vi "AH 2700 Dev Mode.vi"() -> ()   [LabVIEW 2019]
doc: "This example shows how to configure the bridge,initiate deviation mode and continuous capacitance measurement, read the results from the bridge, and parse the measurement results."
uses:
  Andeen-Hagerling 2700(400 firmware).lvlib
panel:
  out "Attentap":string
  out "Voltage":dbl
  out "Loss Greater Than":string
  out "Frequency":dbl
  out "Sample Switch":i32
  in  "Dev Average (s)":dbl=0.1 min=0.0 max=999999.9
  out "Loss Chart":dbl(graph)
  out "Capacitance Chart":dbl(graph)
  in  "Aout Bound\nLower Loss (V)":dbl=-10.0 min=-160.0 max=160.0 format="%#_6f"
  in  "Aout Bound\nLower Cap (V)":dbl=-10.0 min=-160.0 max=160.0 format="%#_6f"
  in  "Aout Bound\nUpper Loss (V)":dbl=10.0 min=-160.0 max=160.0 format="%#_6f"
  in  "Aout Bound\nUpper Cap (V)":dbl=10.0 min=-160.0 max=160.0 format="%#_6f"
  out "Loss":dbl format="%#_10f"
  out "Capacitance":dbl format="%#_10f"
  out "Error Message":string
  in  "Dev Point Loss (jpF)":dbl min=-1900.0 max=19000.0 format="%#_10f"
  in  "Dev Point Cap (pF)":dbl=100.0 min=-165000.0 max=1650000.0 format="%#_10f"
  in  "Deviation Margin":dbl=1.0 min=1.0 max=20.0
  in  "Dev Bound\nLower Loss (jpF)":dbl=-0.1 min=-1900.0 max=19000.0 format="%#_6f"
  in  "Dev Bound\nLower Cap (pF)":dbl=99.0 min=-165000.0 max=1650000.0 format="%#_6f"
  in  "Dev Bound\nUpper Loss (jpF)":dbl=0.1 min=-1900.0 max=19000.0 format="%#_6f"
  in  "Dev Bound\nUpper Cap (pF)":dbl=101.0 min=-165000.0 max=1650000.0 format="%#_6f"
  in  "stop":bool
  in  "Bridge\nFrequency (Hz)":dbl(ring)=1000.0 items=["50"=50.0, "60"=60.0, "70"=70.0, "80"=80.0, "100"=100.0, "120"=120.0, "140"=140.0, "160"=160.0, "200"=200.0, "240"=240.0, "300"=300.0, "400"=400.0, "500"=500.0, "600"=600.0, "700"=700.0, "800"=800.0, "1000"=1000.0, "1200"=1200.0, "1400"=1400.0, "1600"=1600.0, "2000"=2000.0, "2400"=2400.0, "3000"=3000.0, "4000"=4000.0, "5000"=5000.0, "6000"=6000.0, "7000"=7000.0, "8000"=8000.0, "10000"=10000.0, "12000"=12000.0, "14000"=14000.0, "16000"=16000.0, "20000"=20000.0]
  in  "Maximum\nVoltage (V)":dbl=15.0 min=0.0003 max=15.0 step=1.0 format="%#.6f"
  in  "Average\nExponent":u16=4 max=15
  in  "VISA resource":refnum<visa-resource-name>
  in  "Serial Configuration":T1={"Baud Rate"=9600, "Parity"=0, "Data Bits"=8, "Stop Bits"=10} {"Stop Bits" items=["1.0"=10, "1.5"=15, "2.0"=20]; "Data Bits" items=["7"=7, "8"=8]; "Parity" items=["None", "Odd", "Even", "Mark", "Space"]; "Baud Rate" items=["300"=300, "600"=600, "1200"=1200, "2400"=2400, "4800"=4800, "9600"=9600, "19200"=19200, "38400"=38400, "57600"=57600, "115200"=115200]}
  # "AH 2700A ULTRA-PRECISION 50Hz-20kHz CAPACITANCE BRIDGE"
  # "Deviation Mode / Analog Out"
  # "Deviation Parameters"
  # "Measurement Parameters"
  # "Analog Out Parameters"
  # "Measurement Results"
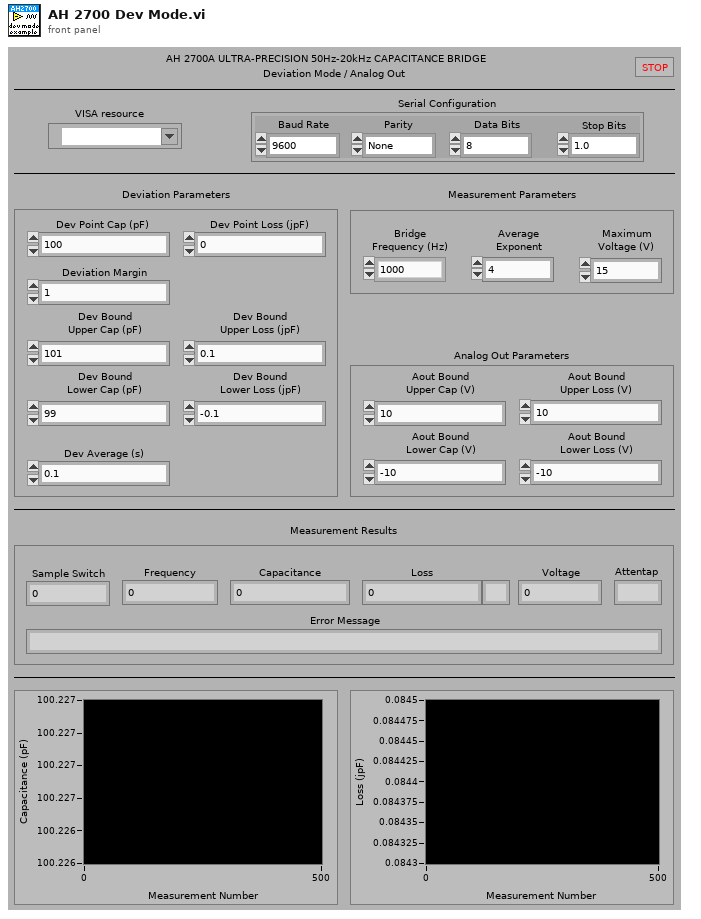
[diagram p1: front panel]
types:
  T1 = cluster{"Baud Rate":u32, "Parity":u16, "Data Bits":u16, "Stop Bits":u16}
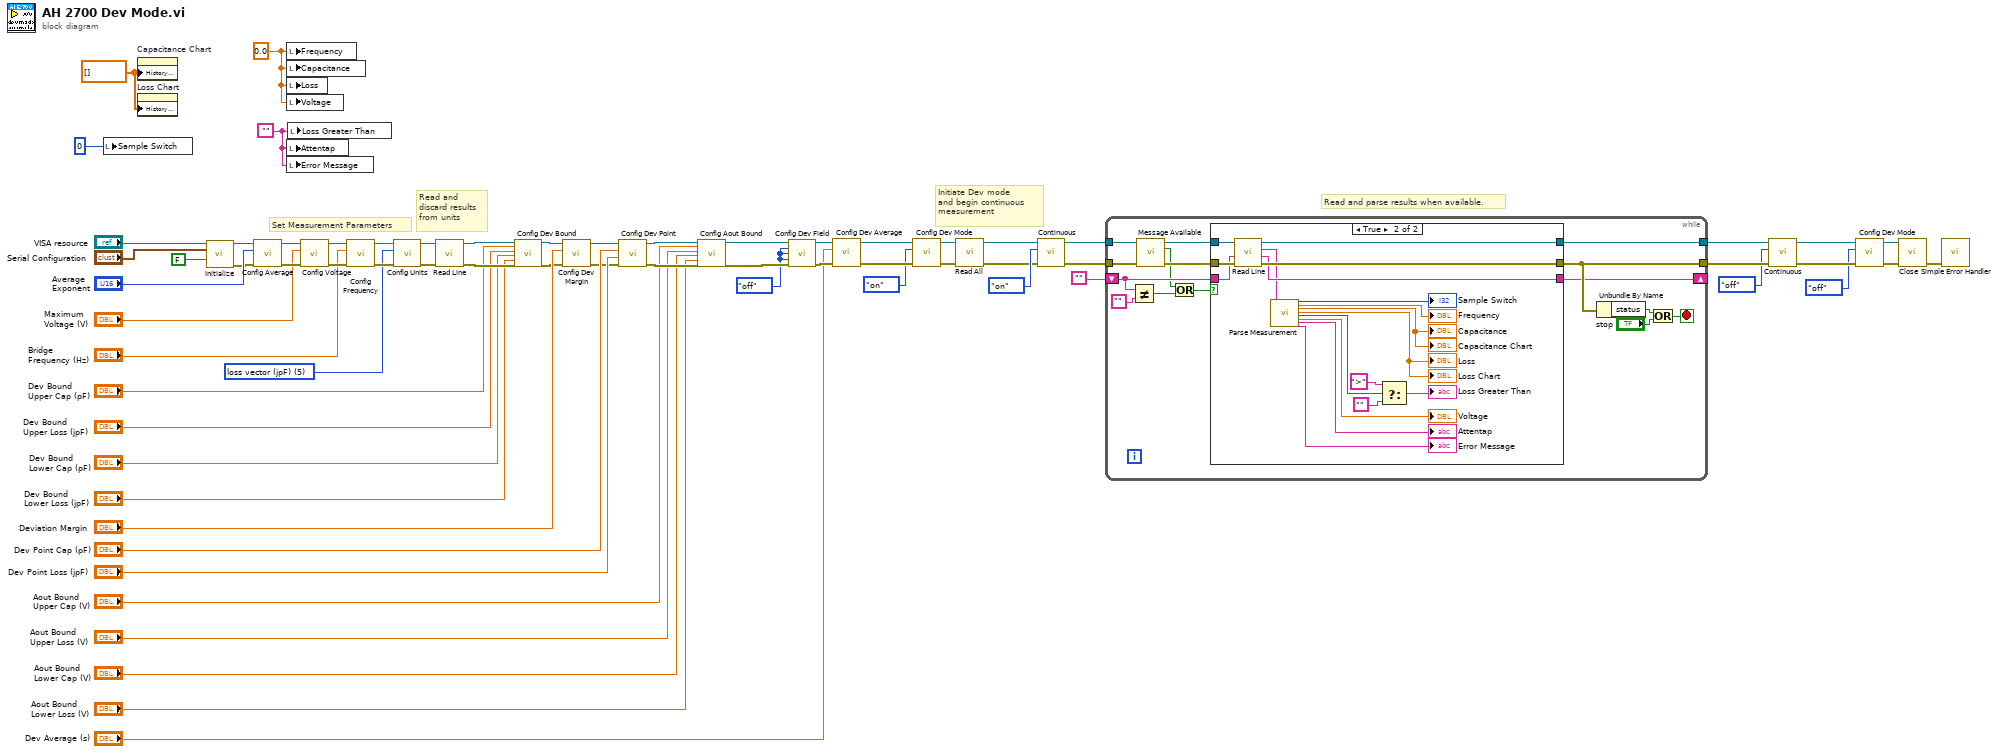
[diagram p0: block diagram]
diagram:
  w1 = ""
  w2 = 0.0 ("Frequency")
  w17 = enum16{"off", "on"}."off" ("Loss (off)")
  w43 = dbl[] [] ("History Data")
  w49 = 5 items=["nanosiemens"=1, "dissipation factor"=2, "kilohms"=3, "gigohms"=4, "loss vector (jpF)"=5] ("Units (nS)")
  # "Read and parse results when available."
  # "Initiate Dev mode\nand begin continuous\nmeasurement"
  # "Set Measurement Parameters"
  # "Read and\ndiscard results\nfrom units"
  n1 = local write "Sample Switch"(0 ("Sample Switch")) -> ()
  n2 = property on="Capacitance Chart" class="WFChart (strict)"("History Data"=w43) -> ()  [unwired: 2 in, 2 out]
  n3 = property on="Loss Chart" class="WFChart (strict)"("History Data"=w43) -> ()  [unwired: 2 in, 2 out]
  n4 = call "Initialize.vi"("VISA resource name"="VISA resource", "Serial Configuration"="Serial Configuration", "Reset (True)"=FALSE) -> ("VISA resource name out"=w35:refnum<visa-resource-name>, "error out"=w34:errorcluster)  [unwired: 11 in]
  n5 = call "Config Average.vi"("error in"=w34, "Average Exponent (4)"="Average\nExponent", "VISA resource name"=w35) -> ("error out"=w63:errorcluster, "VISA resource name out"=w66:refnum<visa-resource-name>)  [unwired: 7 in]
  n6 = local write "Frequency"(w2) -> ()
  n7 = local write "Capacitance"(w2) -> ()
  n8 = local write "Loss"(w2) -> ()
  n9 = local write "Voltage"(w2) -> ()
  n10 = local write "Attentap"(w1) -> ()
  n11 = local write "Error Message"(w1) -> ()
  n12 = local write "Loss Greater Than"(w1) -> ()
  n13 = call "Config Voltage.vi"("error in"=w63, "Voltage (15 V)"="Maximum\nVoltage (V)", "VISA resource name"=w66) -> ("error out"=w62:errorcluster, "VISA resource name out"=w65:refnum<visa-resource-name>)  [unwired: 7 in]
  n14 = call "Config Frequency.vi"("error in"=w62, "Frequency (1000 Hz)"="Bridge\nFrequency (Hz)", "VISA resource name"=w65) -> ("error out"=w61:errorcluster, "VISA resource name out"=w64:refnum<visa-resource-name>)  [unwired: 7 in]
  n15 = call "Config Units.vi"("error in"=w61, "Units (nS)"=w49, "VISA resource name"=w64) -> ("error out"=w56:errorcluster, "VISA resource name out"=w57:refnum<visa-resource-name>)  [unwired: 7 in]
  n16 = call "Read Line.vi"("error in"=w56, "VISA resource name"=w57) -> ("error out"=w32:errorcluster, "VISA resource name out"=w33:refnum<visa-resource-name>)  [unwired: 6 in, 2 out]
  n17 = call "Config Dev Bound.vi"("VISA resource name"=w33, "Upper Capacitance (101 pF)"="Dev Bound\nUpper Cap (pF)", "Upper Loss (0.1 jpF)"="Dev Bound\nUpper Loss (jpF)", "Lower Capacitance (99 pF)"="Dev Bound\nLower Cap (pF)", "Lower Loss (-0.1 jpF)"="Dev Bound\nLower Loss (jpF)", "error in"=w32) -> ("VISA resource name out"=w27:refnum<visa-resource-name>, "error out"=w26:errorcluster)  [unwired: 12 in]
  n18 = call "Config Dev Margin.vi"("error in"=w26, "Margin (1.0)"="Deviation Margin", "VISA resource name"=w27) -> ("error out"=w50:errorcluster, "VISA resource name out"=w51:refnum<visa-resource-name>)  [unwired: 7 in]
  n19 = call "Config Dev Point.vi"("error in"=w50, "Loss (0.0 jpF)"="Dev Point Loss (jpF)", "Capacitance (100.0 pF)"="Dev Point Cap (pF)", "VISA resource name"=w51) -> ("error out"=w24:errorcluster, "VISA resource name out"=w25:refnum<visa-resource-name>)  [unwired: 6 in]
  n20 = call "Config Aout Bound.vi"("VISA resource name"=w25, "Upper Capacitance (10.0 V)"="Aout Bound\nUpper Cap (V)", "Upper Loss (10.0 V)"="Aout Bound\nUpper Loss (V)", "Lower Capacitance (-10.0 V)"="Aout Bound\nLower Cap (V)", "Lower Loss (-10.0 V)"="Aout Bound\nLower Loss (V)", "error in"=w24) -> ("VISA resource name out"=w19:refnum<visa-resource-name>, "error out"=w18:errorcluster)  [unwired: 12 in]
  n21 = call "Config Dev Field.vi"("VISA resource name"=w19, "Counts (off)"=w17, "Capacitance (off)"=w17, "Loss (off)"=w17, "error in"=w18) -> ("VISA resource name out"=w16:refnum<visa-resource-name>, "error out"=w15:errorcluster)  [unwired: 9 in]
  n22 = call "Config Dev Average.vi"("error in"=w15, "Average Time (0.1 sec)"="Dev Average (s)", "VISA resource name"=w16) -> ("error out"=w12:errorcluster, "VISA resource name out"=w13:refnum<visa-resource-name>)  [unwired: 7 in]
  n23 = call "Config Dev Mode.vi"("error in"=w12, "Mode (on)"=enum16{"off", "on"}."on" ("Mode"), "VISA resource name"=w13) -> ("error out"=w9:errorcluster, "VISA resource name out"=w10:refnum<visa-resource-name>)  [unwired: 7 in]
  n24 = call "Read All.vi"("error in"=w9, "VISA resource name"=w10) -> ("error out"=w7:errorcluster, "VISA resource name out"=w6:refnum<visa-resource-name>)  [unwired: 7 in, 1 out]
  n25 = call "Continuous.vi"("error in"=w7, "Scan Measurement (on)"=enum16{"off", "on"}."on", "VISA resource name"=w6) -> ("error out"=w44:errorcluster, "VISA resource name out"=w48:refnum<visa-resource-name>)  [unwired: 7 in]
  n26 = while {
    tunnel: [w78] -> w41
    tunnel: [w77] -> w39
    tunnel: w48 -> [w75]
    tunnel: w44 -> [w73]
    shift-right: [w76] -> _
    shift-left: "" -> [w71]
    stop <- w81 stop-if-true
    n27 = Not Equal?(x=w71, y="") -> (x != y?=w68:bool)
    n28 = call "Message Available.vi"("error in"=w73, "VISA resource name"=w75) -> ("error out"=w72:errorcluster, "message available"=w67:bool, "VISA resource name out"=w74:refnum<visa-resource-name>)  [unwired: 7 in]
    n29 = Or(x=w67, y=w68) -> (x .or. y?=w69:bool)
    n30 = case shown="True" w69 {
      tunnel: [w84 w102] -> w78
      tunnel: [w83 w101] -> w77
      tunnel: [w82 w97] -> w76
      tunnel: w71 -> [w82 w98]
      tunnel: w74 -> [w84 w100]
      tunnel: w72 -> [w83 w99]
      frame False {
      }
      frame True {
        n31 = call "Read Line.vi"("error in"=w99, "Previous"=w98, "VISA resource name"=w100) -> ("error out"=w101:errorcluster, "Remaining"=w97:string, "Message"=w96:string, "VISA resource name out"=w102:refnum<visa-resource-name>)  [unwired: 5 in]
        n32 = call "Parse Measurement.vi"("Measurement Line"=w96) -> ("Sample"=→"Sample Switch":i32, "Frequency"=→"Frequency":dbl, "Capacitance"=→"Capacitance" →"Capacitance Chart":dbl, "Loss"=→"Loss" →"Loss Chart":dbl, "Loss Greater Than"=w91:bool, "Voltage"=→"Voltage":dbl, "Attentap"=→"Attentap":string, "Error Message"=→"Error Message":string)  [unwired: 17 in, 2 out]
        n33 = Select(t=">", s=w91, f="") -> (s? t:f=→"Loss Greater Than":string)
      }
    }
    n34 = Unbundle By Name(w77) -> ("status"=w80:bool)
    n35 = Or(x=w80, y="stop") -> (x .or. y?=w81:bool)
  }
  n36 = call "Continuous.vi"("error in"=w39, "Scan Measurement (on)"=enum16{"off", "on"}."off", "VISA resource name"=w41) -> ("error out"=w40:errorcluster, "VISA resource name out"=w42:refnum<visa-resource-name>)  [unwired: 7 in]
  n37 = call "Config Dev Mode.vi"("error in"=w40, "Mode (on)"=enum16{"off", "on"}."off" ("Mode"), "VISA resource name"=w42) -> ("error out"=w45:errorcluster, "VISA resource name out"=w46:refnum<visa-resource-name>)  [unwired: 7 in]
  n38 = call "Close.vi"("error in (no error)"=w45, "VISA resource name"=w46) -> ("error out"=w55:errorcluster)  [unwired: 9 in]
  n39 = call <vilib>:"Simple Error Handler.vi"("error in (no error)"=w55) -> ()  [unwired: 4 in, 5 out]
